vi "Init.vi"(8 "error in (no error)":errorcluster caption="entrée d'erreur (pas d'erreur)", 11 "Class UART Nodon.lvclass En entrée":refnum<class "Class UART Zigbee.lvclass">) -> (0 "error out":errorcluster caption="sortie d'erreur", 3 "Class UART Nodon.lvclass En sortie":refnum<class "Class UART Zigbee.lvclass">)   [LabVIEW 2020, in "Library Instrument & Equipement.lvlib" / "Library UART.lvlib" / "Class UART Zigbee.lvclass"]
uses:
  Class UART Zigbee.lvclass
  C:/Users/ngarcin/OneDrive - Altyor/Standard TB/Class/UART/UART (Default)/Class UART (Default).lvclass
  UART (Default)/Class UART (Default).lvclass
  Class UART Zigbee.lvclass/Class UART Zigbee.ctl
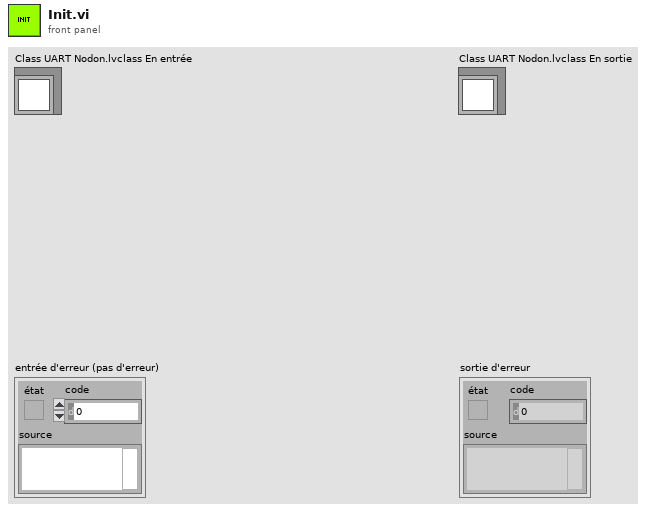
[diagram p1: front panel]
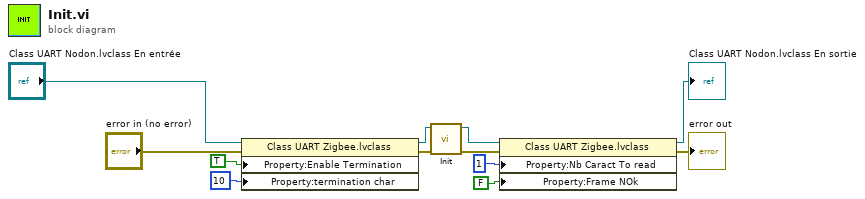
[diagram p0: block diagram]
diagram:
  n1 = property class="Class UART Zigbee.lvclass"(reference="Class UART Nodon.lvclass En entrée", error in="error in (no error)", "Property:Enable Termination"=TRUE ("Enable Termination"), "Property:termination char "=u8 10 ("termination char")) -> (reference out=w5:refnum<class "Class UART Zigbee.lvclass">, error out=w3:errorcluster)
  n2 = call-parent "Init.vi"("error in (no error)"=w3, "Class UART (Default) en entrée"=w5) -> ("error out"=w11:errorcluster, "Class UART (Default) en sortie"=w10:refnum<class "Class UART Zigbee.lvclass">)  [unwired: 8 in]
  n3 = property class="Class UART Zigbee.lvclass"(reference=w10, error in=w11, "Property:Nb Caract To read"=u32 1 ("Nb Caract To read"), "Property:Frame NOk"=FALSE ("Frame NOk")) -> (reference out=→"Class UART Nodon.lvclass En sortie":refnum<class "Class UART Zigbee.lvclass">, error out=→"error out":errorcluster)
